vi "Autotest_Instr.vi"(8 "error in (no error)":errorcluster caption="entrée d'erreur (pas d'erreur)", 11 "Class Instrument Multimeter en entrée":refnum<class "Class Instrument LED_Analyser.lvclass">) -> (0 "error out":errorcluster caption="sortie d'erreur", 3 "Class Instrument Multimeter en sortie":refnum<class "Class Instrument LED_Analyser.lvclass">)   [LabVIEW 2020, in "Library Instrument & Equipement.lvlib" / "Library Instruments.lvlib" / "Class Instrument LED_Analyser.lvclass"]
uses:
  Class Instrument LED_Analyser.lvclass
  C:/Users/ngarcin/OneDrive - Altyor/Standard TB/Class/Instrument/Instrument (Default)/Class Instrument (Default).lvclass
  Class Instrument LED_Analyser.lvclass/Class Instrument LED_Analyser.ctl
  Instrument (Default)/Class Instrument (Default).lvclass
  LED Analyser/Class Led Analyser (Default)/Class LED Analyser (Default).lvclass
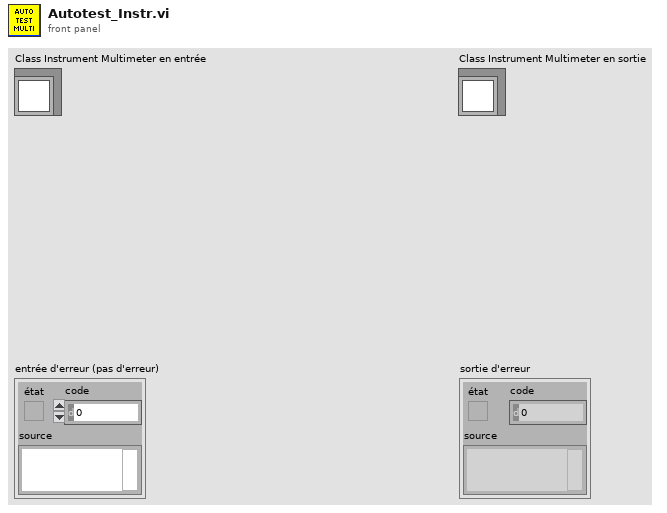
[diagram p1: front panel]
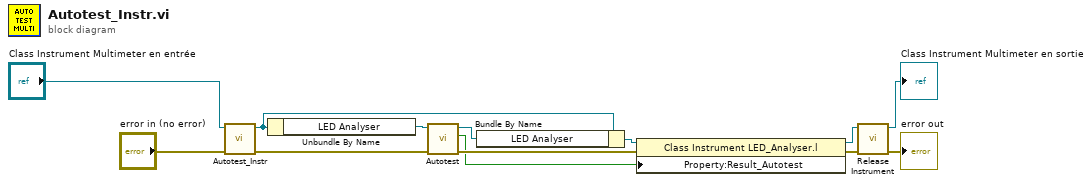
[diagram p0: block diagram]
diagram:
  n1 = call-parent "Autotest_Instr.vi"("error in (no error)"="error in (no error)", "Class Instrument (Default) en entrée"="Class Instrument Multimeter en entrée") -> ("error out"=w5:errorcluster, "Class Instrument (Default) en sortie"=w11:refnum<class "Class Instrument LED_Analyser.lvclass">)  [unwired: 8 in]
  n2 = Unbundle By Name(w11) -> ("LED Analyser"=w3:refnum<class "Class LED Analyser (Default).lvclass">)
  n3 = call-dynamic "Autotest.vi"("error in (no error)"=w5, "Class LED Analyser in"=w3) -> ("error out"=w4:errorcluster, "Autotest Ok ?"=w2:bool, "Class LED Analyser Out"=w1:refnum<class "Class LED Analyser (Default).lvclass">)  [unwired: 7 in]
  n4 = Bundle By Name(cluster=w11, "LED Analyser"=w1) -> (w10:refnum<class "Class Instrument LED_Analyser.lvclass">)
  n5 = property class="Class Instrument LED_Analyser.l"(reference=w10, error in=w4, "Property:Result_Autotest"=w2) -> (reference out=w7:refnum<class "Class Instrument LED_Analyser.lvclass">, error out=w9:errorcluster)
  n6 = call-dynamic "Release Instrument.vi"("error in (no error)"=w9, "Class Instrument (Default) en entrée"=w7) -> ("error out"=→"error out":errorcluster, "Class Instrument (Default) en sortie"=→"Class Instrument Multimeter en sortie":refnum<class "Class Instrument LED_Analyser.lvclass">)  [unwired: 8 in]
